vi "PH_Sequencer.PC Action PPMAStateSM.vi"(0 "i ref in":refnum<vi>, 5 "error in (no error)":errorcluster) -> (14 "i ref out":refnum<vi>, 19 "error out":errorcluster)   [LabVIEW 2014, in "PH_Sequencer.lvlib"]
doc: "This is the action of the case PPMAStateSM: depending on the state, it dis- or enbles the set voltage element and writes to GUI and own attributes, if the PUs of the PPMA are running."
uses:
  PH_Sequencer.lvlib
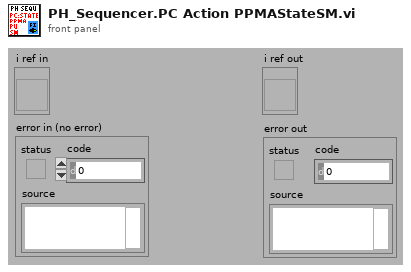
[diagram p1: front panel]
types:
  T1 = typedef "PH_Sequencer.lvlib/PH_Sequencer.i attribute.ctl" = cluster{"GUI Refs":cluster{"Main Off":refnum<vi>, "Fire":refnum<vi>, "Status":refnum<vi>, "Ready":refnum<vi>, "Waiting Time":refnum<vi>, "Timeout":refnum<vi>, "PPMA Ready":refnum<vi>, "Sequencer SM State":refnum<vi>, "PPPA Ready":refnum<vi>, "Calorimeter":refnum<vi>, "Beamline Ready":refnum<vi>, "Clear Beamline":refnum<vi>, "Linkage PPMA Rods":refnum<vi>, "Linkage Current PA":refnum<vi>, "Linkage Current MA":refnum<vi>, "Timing Ready":refnum<vi>, "State Timing":refnum<vi>, "Force Timing":refnum<vi>, "PSDB Shot Comment":refnum<vi>, "State PA Backreflection":refnum<vi>, "Beamline Z6 Ready":refnum<vi>, "Clear Z6 Beamline":refnum<vi>, "Sequence length":refnum<vi>, "Timing Mode":refnum<vi>, "Slow Trigger Settings":refnum<vi>, "Experiment Description":refnum<vi>, "State PSDB":refnum<vi>, "PSDB Ready":refnum<vi>, "Set PSDB Settings":refnum<vi>, "Get PSDB Info":refnum<vi>, "Take Snapshot":refnum<vi>, "Shottype":refnum<vi>, "Experiment":refnum<vi>, "Phase Frontends":refnum<vi>}, "Status Info":cluster{"Machine Status":T2, "WaitingTime":i32, "Timeout":bool}, "Readyness":cluster{"Ready to shot":bool, "PPMA Ready":bool, "PPPA Ready":bool, "BL Ready":bool, "Timing Ready":bool, "BL Z6 Ready":bool, "PSDBReady":bool}, "Instancenames":cluster{"PPMA Rods":string, "PP Current Meas":string, "Beamline":string, "PA Backrefl Meas":string, "Beamline Z6":string}, "Data to read":bool, "Calorimeter":cluster{"Instancename":string, "On":bool, "linked":bool}, "Linkage":cluster{"PPMA Rods":bool, "PP Current Meas":bool, "Beamline":bool, "PA Backrefl Meas":bool, "Beamline Z6":bool}, "Timing":cluster{"Instance":string, "linked":bool, "Status":T2, "Timing Mode":T3, "Slow Trigger Settings":T4, "Info available":cluster{"ext SlowTrigger":bool, "T2":bool, "Mode":bool, "Delay Slow Trigger":bool, "Phase FEs":bool}, "FE Phase":T5}, "Service ID R2S":i32, "PSDB":cluster{"Controller Instance":string, "Controller Status":T2, "Controller linked":bool, "Settings acknowledged":bool, "Current Experiment ID":i16, "Current Shot Type":i16, "Current Comment":string, "Remember Settings":bool, "Write 2 early":bool}, "PSDB Data":cluster{"Main Off?":bool, "Sequence Length":dbl, "Sequence startet":timestamp}, "6P 4Q Positions":cluster{"Instancename":string, "linked":bool, "Position":T6}[], "PUs":T7[], "PPMA PUs":cluster{"PowerUnit":T8, "GUI Ref":refnum<vi>, "PPMA PU Information":T10}[], "PPPA PUs":cluster{"PowerUnit":T8, "GUI Ref":refnum<vi>, "PPPA PU Information":T11}[]}
  T2 = typedef "Status.ctl" = i16
  T3 = typedef "PH_Timing.lvlib/PH_Timing.Timing Mode.ctl" = cluster{"T2":i16, "Modeselector":enum32{"10 Hz", "0.5 Hz", "Shot"}}
  T4 = typedef "PH_Timing.lvlib/PH_Timing.Slow Trigger Settings.ctl" = cluster{"Delay":dbl, "externally triggered?":bool}
  T5 = typedef "PH_Timing.lvlib/PH_Timing.Phase FEs.ctl" = cluster{"Phase":dbl}
  T6 = typedef "PH_4_Pos_Selector.lvlib/PH_4_Pos_Selector.Position Selector.ctl" = u16
  T7 = typedef "PH_Sequencer.lvlib/PH_Sequencer.Head.ctl" = cluster{"PowerUnit":T8, "GUI Ref":refnum<vi>, "Information":T9, "linked?":bool}
  T8 = typedef "PH_Common.PP PUs.ctl" = enum16{"no Info", "PA-19mm-1", "PA-19mm-2", "PA-45mm-PILC", "PA-45mm-MAIN", "MA-PU-1", "MA-PU-2", "MA-PU-3", "MA-PU-4", "MA-PU-5", "MA-PU-6", "MA-FR", "MA-PILC", "PA-45mm-DP"}
  T9 = typedef "PH_Sequencer.lvlib/PH_Sequencer.PU Information.ctl" = cluster{"State":T2, "Waiting Time [s]":dbl, "R2S?":bool, "GD CH on?":bool, "Shot over?":bool}
  T10 = typedef "PH_Sequencer.lvlib/PH_Sequencer.PPMA PU Information.ctl" = cluster{"Current Voltage [V]":dbl, "PU State SM":string, "PU Timeout SM":string, "Rods Up?":bool}
  T11 = typedef "PH_Sequencer.lvlib/PH_Sequencer.PPPA PU Information.ctl" = cluster{"Current Voltage [V]":dbl, "PU State SM":string, "PU Timeout SM":string, "Close RR?":bool}
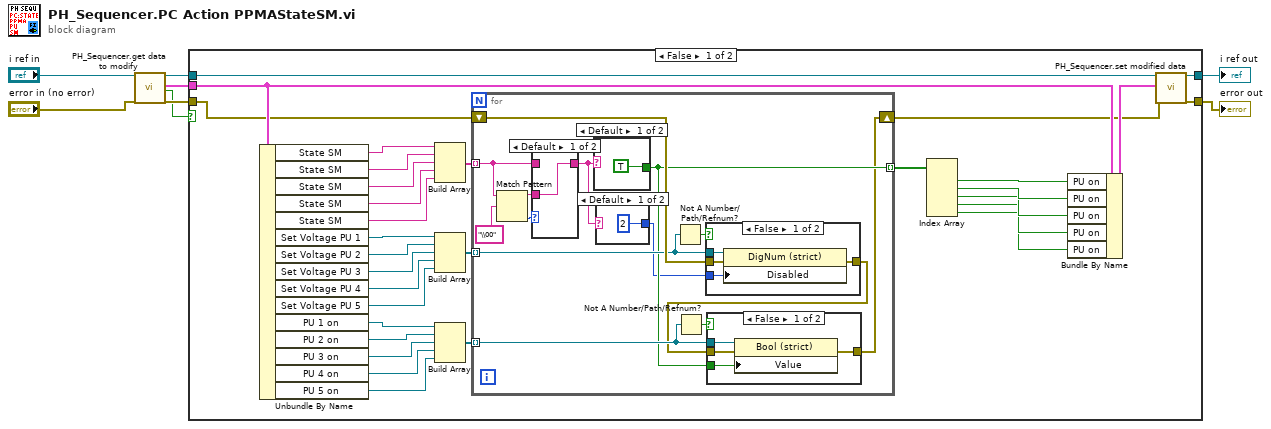
[diagram p0: block diagram]
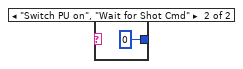
[diagram p3: hidden frame]
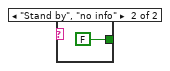
[diagram p5: hidden frame]
diagram:
  n1 = call "PH_Sequencer.get data to modify.vi"("i ref in"="i ref in", "error in (no error)"="error in (no error)") -> ("i ref out"=w4:refnum<vi>, "i attribute"=w2:T1, "timed out"=w1:bool, "error out"=w3:errorcluster)  [unwired: 14 in]
  n2 = case shown="False" w1 {
    tunnel: [w38 w71] -> w8
    tunnel: [w37 w70] -> w6
    tunnel: w4 -> [w36 w71]
    tunnel: w3 -> [w10 w70]
    tunnel: w2 -> [w35 _]
    frame False {
      n3 = Unbundle By Name(w35) -> ("State SM"=w29:string, "State SM"=w28:string, "State SM"=w27:string, "State SM"=w26:string, "State SM"=w25:string, "Set Voltage PU 1"=w34:refnum<vi>, "Set Voltage PU 2"=w33:refnum<vi>, "Set Voltage PU 3"=w32:refnum<vi>, "Set Voltage PU 4"=w31:refnum<vi>, "Set Voltage PU 5"=w30:refnum<vi>, "PU 1 on"=w22:refnum<vi>, "PU 2 on"=w21:refnum<vi>, "PU 3 on"=w20:refnum<vi>, "PU 4 on"=w19:refnum<vi>, "PU 5 on"=w18:refnum<vi>)
      n4 = Build Array(w29, w28, w27, w26, w25) -> (w23:string[])
      n5 = Build Array(w34, w33, w32, w31, w30) -> (w24:refnum<vi>[])
      n6 = Build Array(w22, w21, w20, w19, w18) -> (w17:refnum<vi>[])
      n7 = for {
        tunnel: w24 -> [w48] mode=indexing
        shift-right: [w46] -> w9
        shift-left: w10 -> [w53]
        tunnel: w23 -> [w41] mode=indexing
        tunnel: [w47] -> w11 mode=indexing
        tunnel: w17 -> [w50] mode=indexing
        n8 = Match Pattern(string=w41, regular expression="\\00" ("search string")) -> (before substring=w43:string, offset past match=w42:i32)  [unwired: 1 in, 2 out]
        n9 = case shown="Default" w42 {
          tunnel: [w54 w55] -> w40
          tunnel: w41 -> [_ w55]
          tunnel: w43 -> [w54 _]
          frame Default {
          }
          frame -1 {
          }
        }
        n10 = case shown="Default" w40 {
          tunnel: [TRUE FALSE] -> w47
          frame Default {
          }
          frame "Stand by", "no info" {
          }
        }
        n11 = case shown="Default" w40 {
          tunnel: [2 0] -> w45
          frame Default {
          }
          frame "Switch PU on", "Wait for Shot Cmd" {
          }
        }
        n12 = Not A Number/Path/Refnum?(number/path/refnum=w48) -> (NaN/Path/Refnum?=w52:bool)
        n13 = Not A Number/Path/Refnum?(number/path/refnum=w50) -> (NaN/Path/Refnum?=w51:bool)
        n14 = case shown="False" w52 {
          tunnel: w48 -> [w68 _]
          tunnel: w53 -> [w67 w69]
          tunnel: [w66 w69] -> w49
          tunnel: w45 -> [w65 _]
          frame False {
            n15 = property class="DigNum (strict)"(reference=w68, error in=w67, "Disabled"=w65) -> (error out=w66:errorcluster)  [unwired: 1 out]
          }
          frame True {
          }
        }
        n16 = case shown="False" w51 {
          tunnel: w50 -> [w61 _]
          tunnel: w49 -> [w60 w62]
          tunnel: [w59 w62] -> w46
          tunnel: w47 -> [w58 _]
          frame False {
            n17 = property class="Bool (strict)"(reference=w61, error in=w60, "Value"=w58) -> (error out=w59:errorcluster)  [unwired: 1 out]
          }
          frame True {
          }
        }
      }
      n18 = Index Array(array=w11) -> (element #1=w16:bool, element #2=w15:bool, element #3=w14:bool, element #4=w13:bool, element #5=w12:bool)  [unwired: 5 in]
      n19 = Bundle By Name(cluster=w35, "PU on"=w16, "PU on"=w15, "PU on"=w14, "PU on"=w13, "PU on"=w12) -> (w39:T1)
      n20 = call "PH_Sequencer.set modified data.vi"("i ref in"=w36, "i attribute"=w39, "error in (no error)"=w9) -> ("i ref out"=w38:refnum<vi>, "error out"=w37:errorcluster)  [unwired: 15 in]
    }
    frame True {
    }
  }
  "i ref out" <- w8
  "error out" <- w6
